vi "StartMeasurement.vi"(8 "error in (no error)":errorcluster, 11 "object in":refnum<class "Tesla Tester GUI.lvclass">) -> (0 "error out":errorcluster, 3 "object out":refnum<class "Tesla Tester GUI.lvclass">)   [LabVIEW 2013, in "Tesla Tester GUI.lvlib" / "Tesla Tester GUI.lvclass"]
uses:
  Tesla Tester GUI.lvclass
  Tesla Tester GUI.lvclass/Tesla Tester GUI.ctl
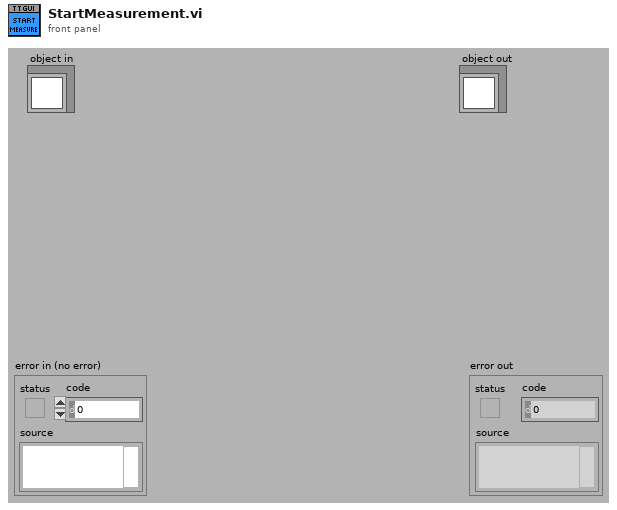
[diagram p1: front panel]
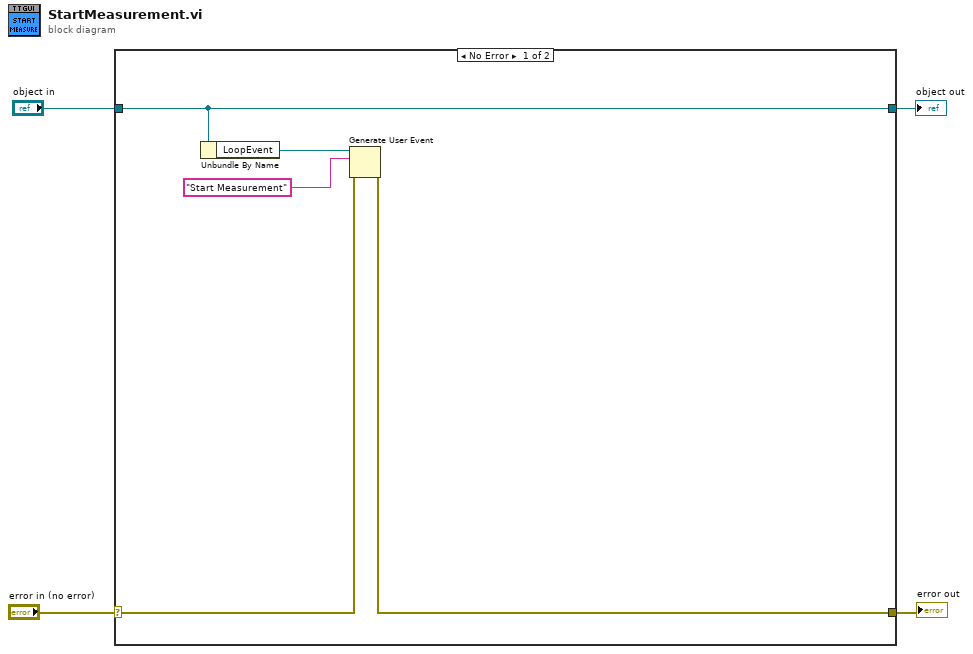
[diagram p0: block diagram]
diagram:
  n1 = case shown="No Error" "error in (no error)" {
    selector: "error in (no error)" -> [w7 w11]
    tunnel: [w6 w11] -> w3
    tunnel: [w9 w10] -> w1
    tunnel: "object in" -> [w9 w10]
    frame No Error {
      n2 = Unbundle By Name(w9) -> ("LoopEvent"=w8:refnum<user-event>)
      n3 = Generate User Event(user event=w8, event data cluster="Start Measurement", error in=w7) -> (error out=w6:errorcluster)  [unwired: 1 in, 1 out]
    }
    frame Error {
    }
  }
  "error out" <- w3
  "object out" <- w1
